vi "DUAL GAUGE-Sensor Identify.vi"(8 "Fehler (Eingang)":errorcluster, 11 "Referenz in":refnum<visa-resource-name>) -> (0 "Cluster (Ausgang)":errorcluster, 1 "Sensor 2":string, 2 "Sensor 1":string, 3 "Referenz out":refnum<visa-resource-name>)   [LabVIEW 2017, in "Dual Gauge.lvlib"]
uses:
  <userlib>/Dual Gauge/Dual Gauge.lvlib
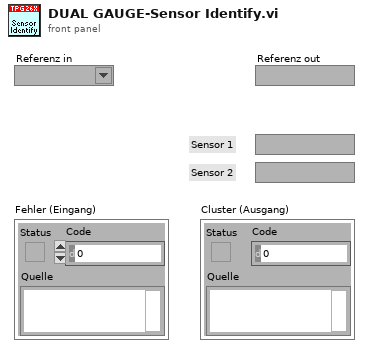
[diagram p1: front panel]
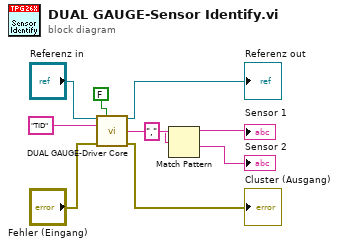
[diagram p0: block diagram]
diagram:
  n1 = call <userlib>:"DUAL GAUGE-Driver Core.vi"("Referenz in"="Referenz in", "Write/Read"=FALSE, "Command"="TID", "Fehler (Eingang)"="Fehler (Eingang)") -> ("Referenz out"=→"Referenz out":refnum<visa-resource-name>, "String Out"=w8:string, "Cluster (Ausgang)"=→"Cluster (Ausgang)":errorcluster)  [unwired: 9 in]
  n2 = Match Pattern(string=w8, regular expression="," ("search char (-)")) -> (before substring=→"Sensor 1":string, after substring=→"Sensor 2":string)  [unwired: 1 in, 2 out]
